vi "operation.vi"() -> ()   [LabVIEW 2020]
panel:
  in  "Tab Control":enum32{"Page 1", "Page 2"}(tab)
  in  "Next Button":bool
  in  "sum":bool
  out "output 4":dbl
  in  "input 6":dbl
  in  "input 5":dbl
  in  "stop 2":bool
  in  "Previous Button":bool
  out "Boolean 2":bool
  in  "Boolean":bool
  in  "input 4":dbl
  out "output 3":dbl
  in  "input 3":dbl
  in  "stop":bool
  in  "input 2":dbl
  out "output 2":dbl
  in  "input 1":dbl
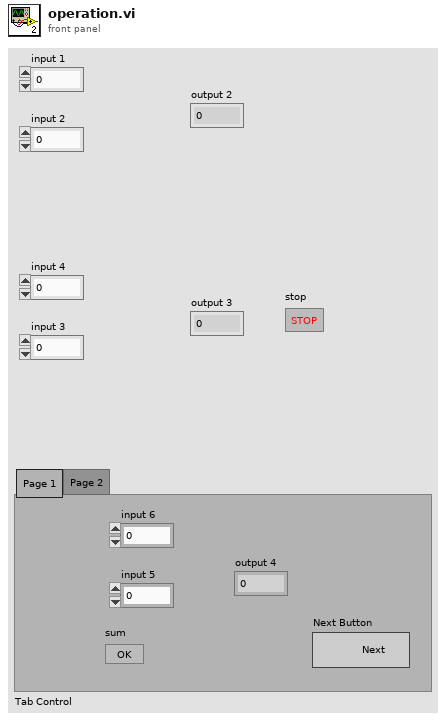
[diagram p1: front panel]
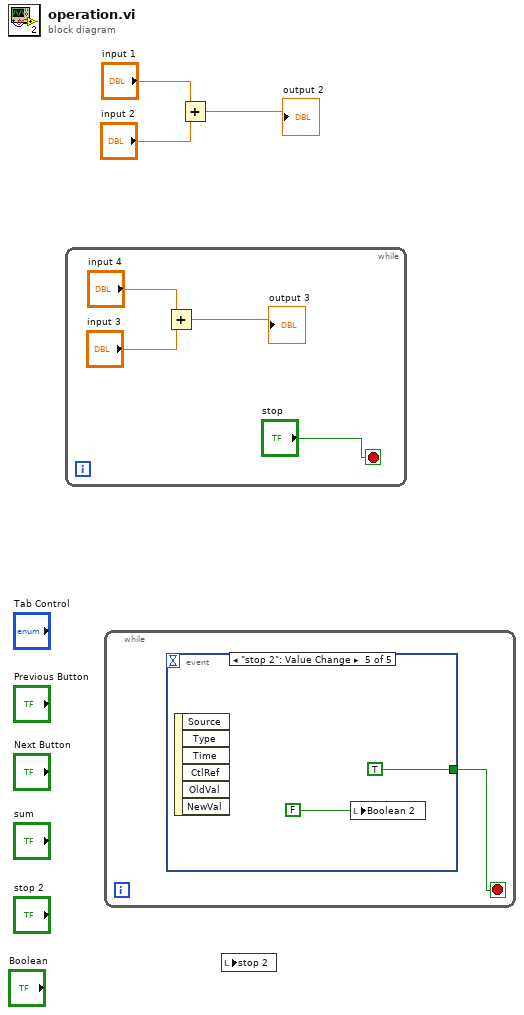
[diagram p0: block diagram]
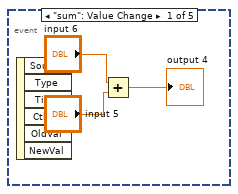
[diagram p2: hidden frame]
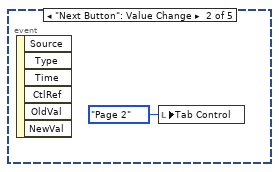
[diagram p3: hidden frame]
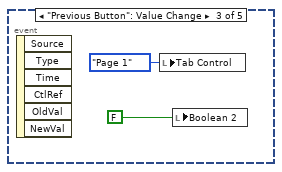
[diagram p4: hidden frame]
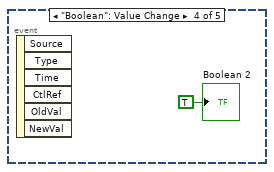
[diagram p5: hidden frame]
diagram:
  n1 = while {
    stop <- "stop" stop-if-true
    n2 = Add(x="input 3", y="input 4") -> (x+y=→"output 3":dbl)
  }
  n3 = while {
    stop <- w8 stop-if-true
    n4 = event shown="[4] \"stop 2\": Value Change" {
      selector: _ -> [_ _ _ _ _]
      dyn-events: _ -> [_ _ _ _ _]
      timeout: _ -> [_ _ _ _ _]
      tunnel: [_ _ _ _ TRUE] -> w8
      event "sum": Value Change {
        n5 = event-data() -> ()  [unwired: 1 in, 6 out]
        n6 = Add(x="input 6", y="input 5") -> (x+y=→"output 4":dbl)
      }
      event "Next Button": Value Change {
        n7 = event-data() -> ()  [unwired: 1 in, 6 out]
        n8 = local write "Tab Control"(enum32{"Page 1", "Page 2"}."Page 2" ("Tab Control")) -> ()
      }
      event "Previous Button": Value Change {
        n9 = event-data() -> ()  [unwired: 1 in, 6 out]
        n10 = local write "Tab Control"(enum32{"Page 1", "Page 2"}."Page 1" ("Tab Control")) -> ()
        n11 = local write "Boolean 2"(FALSE ("Boolean 2")) -> ()
      }
      event "Boolean": Value Change {
        n12 = event-data() -> ()  [unwired: 1 in, 6 out]
        "Boolean 2" <- TRUE ("Boolean 2")
      }
      event "stop 2": Value Change {
        n13 = event-data() -> ()  [unwired: 1 in, 6 out]
        n14 = local write "Boolean 2"(FALSE ("Boolean 2")) -> ()
      }
    }
  }
  n15 = Add(x="input 1", y="input 2") -> (x+y=→"output 2":dbl)
  n16 = local read "stop 2"() -> ()  [unwired: 1 in]
